vi "Data2StatID.vi"(10 "ParameterSet":string, 11 "Step":string) -> (3 "StatID":string)   [LabVIEW 2013]
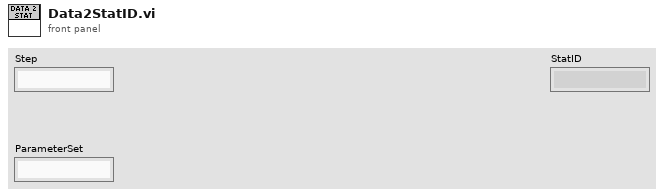
[diagram p1: front panel]
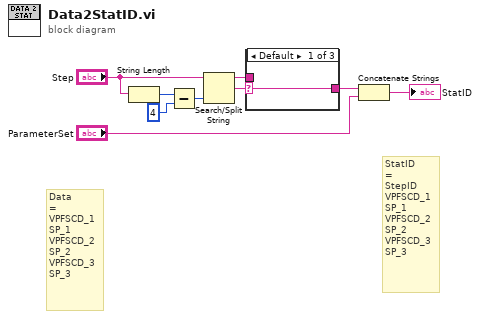
[diagram p0: block diagram]
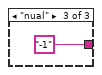
[diagram p3: hidden frame]
diagram:
  # "StatID\n=\nStepID\nVPFSCD_1\nSP_1\nVPFSCD_2\nSP_2\nVPFSCD_3\nSP_3"
  # "Data\n=\nVPFSCD_1\nSP_1\nVPFSCD_2\nSP_2\nVPFSCD_3\nSP_3"
  n1 = String Length(string="Step") -> (length=w8:i32)
  n2 = Subtract(x=w8, y=4) -> (x-y=w5:i32)
  n3 = Search/Split String(string="Step", offset (0)=w5) -> (substring before match=w4:string, match + rest of string=w6:string)  [unwired: 1 in, 1 out]
  n4 = case shown="Default" w6 {
    selector: w6 -> [w10 _ _]
    tunnel: [w10 w11 "-1"] -> w3
    tunnel: w4 -> [_ w11 _]
    frame Default {
    }
    frame " (M)" {
    }
    frame "nual" {
    }
  }
  n5 = Concatenate Strings(w3, "ParameterSet") -> (→"StatID":string)
